vi "Load (1).vi"(4 "Tare":bool, 5 "Excitation Voltage (in Volt)":dbl=10.0, 6 "Maximum Load (in Kg)":dbl=50.0, 7 "Sensitivity (in Volt)":dbl=2.0, 8 "error in (no error)":errorcluster, 11 "Load In Volt":dbl) -> (0 "error out":errorcluster, 3 "Load (kg)":dbl)   [LabVIEW 2021]
uses:
  <vilib>/Utility/config.llb/Write Key (Double).vi
  <vilib>/Utility/config.llb/NI_LVConfig.lvlib
panel:
  out "Load Tare Value":dbl
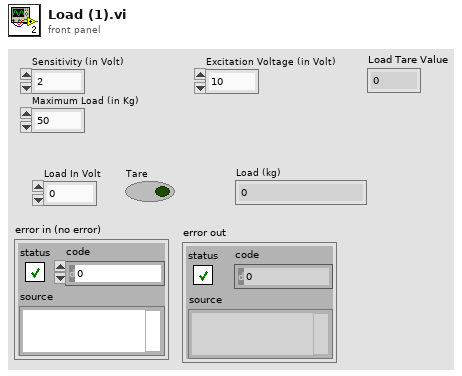
[diagram p1: front panel]
types:
  T1 = typedef "NI_LVConfig.lvlib/Config Data RefNum.ctl" = refnum<k1>
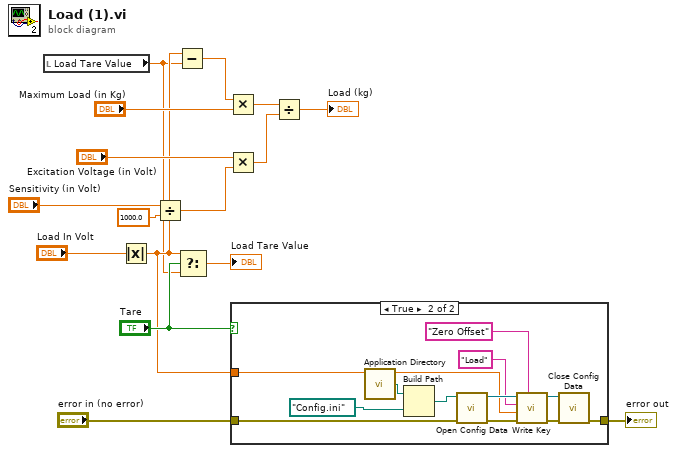
[diagram p0: block diagram]
diagram:
  n1 = local read "Load Tare Value"() -> (w3:dbl)
  n2 = Absolute Value(x="Load In Volt") -> (abs(x)=w6:dbl)
  n3 = Divide(x="Sensitivity (in Volt)", y=1000.0) -> (x/y=w13:dbl)
  n4 = Subtract(x=w6, y=w3) -> (x-y=w5:dbl)
  n5 = Select(t=w6, s="Tare", f=w3) -> (s? t:f=→"Load Tare Value":dbl)
  n6 = Multiply(x=w5, y="Maximum Load (in Kg)") -> (x*y=w16:dbl)
  n7 = Multiply(x="Excitation Voltage (in Volt)", y=w13) -> (x*y=w15:dbl)
  n8 = case shown="True" "Tare" {
    tunnel: w6 -> [_ w23]
    tunnel: "error in (no error)" -> [w17 w22]
    tunnel: [w17 w21] -> w1
    frame False {
    }
    frame True {
      n9 = call <vilib>:"Application Directory.vi"() -> ("Application Directory"=w20:path)
      n10 = Build Path(base path=w20, name or relative path=path "Config.ini" ("default name")) -> (appended path=w18:path)
      n11 = call <vilib>:"Open Config Data.vi"("error in (no error)"=w22, "configuration file path"=w18) -> ("error out"=w27:errorcluster, "refnum"=w29:T1)  [unwired: 7 in, 1 out]
      n12 = call-poly <vilib>:"Write Key.vi"("section"="Zero Offset", "error in (no error)"=w27, "value"=w23, "key"="Load", "refnum"=w29) -> ("error out"=w26:errorcluster, "refnum out"=w28:T1)  [unwired: 4 in, 1 out]
      n13 = call <vilib>:"Close Config Data.vi"("error in (no error)"=w26, "refnum"=w28) -> ("error out"=w21:errorcluster)  [unwired: 8 in, 1 out]
    }
  }
  "error out" <- w1
  n14 = Divide(x=w16, y=w15) -> (x/y=→"Load (kg)":dbl)
